vi "CRYGet BroadBand Curve.vi"(9 "Unit Info In":T5={"Y unit In"="dB", "dB ref In"=1.0, "Y unit Out"="dB", "dB ref Out"=1.0, "Y unit Curve"="dB", "dB ref Curve"=1.0, "Y data  Curve"=0, "Y data Time"=0}, 10 "Additive Info":T3, 11 "Impedance and Mic Current In":bool[](array[boolean])) -> (1 "Display Array":T4(array[cluster]), 2 "Unit Info Out":T2[](array[typedef]), 3 "Curve Info Array Out":T1)   [LabVIEW 2013]
uses:
  Typedef Control/CRYUnit Info Cluster.ctl
  Typedef Control/CRYUnit Info Out Cluster.ctl
  Typedef Control/CRYAnalysis CurveName Cluster.ctl
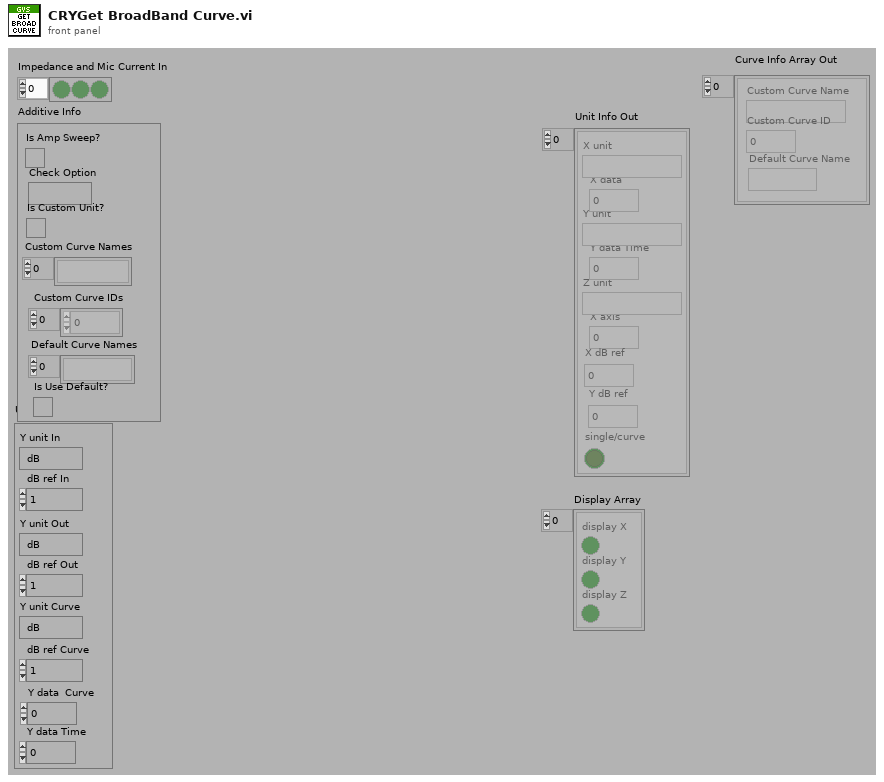
[diagram p1: front panel]
types:
  T1 = typedef "CRYAnalysis CurveName Cluster.ctl" = cluster{"Custom Curve Name":string, "Custom Curve ID":i32, "Default Curve Name":string}[]
  T2 = typedef "CRYUnit Info Out Cluster.ctl" = cluster{"X unit":string, "X data":u16, "Y unit":string, "Y data Time":u16, "Z unit":string, "X axis":u16, "X dB ref":dbl, "Y dB ref":dbl, "single/curve":bool}
  T3 = cluster{"Is Amp Sweep?":bool, "Check Option":string, "Is Custom Unit?":bool, "Custom Curve Names":string[], "Custom Curve IDs":i32[], "Default Curve Names":string[], "Is Use Default?":bool}
  T4 = cluster{"display X":bool, "display Y":bool, "display Z":bool}[]
  T5 = typedef "CRYUnit Info Cluster.ctl" = cluster{"Y unit In":string, "dB ref In":dbl, "Y unit Out":string, "dB ref Out":dbl, "Y unit Curve":string, "dB ref Curve":dbl, "Y data  Curve":u16, "Y data Time":u16}
  T6 = cluster{"display X":bool, "display Y":bool, "display Z":bool}
  T7 = enum32{"English", "Chinese", "Korean", "Japanese", "Russian", "Chinese traditional"}
  T8 = cluster{"Y unit Out":string, "dB":u16, "Y unit Curve":string, "Y data  Curve":u16, "Y unit Curve":string, "Lin":u16, "dB ref Out":dbl, "dB ref Curve":dbl, "display X":bool}
  T9 = cluster{"Y unit Out":string, "dB":u16, "Y unit Curve":string, "Y data  Curve":u16, "Y unit Curve":string, "Lin":u16, "dB ref Out":dbl, "dB ref Curve":dbl, "display X":bool}[]
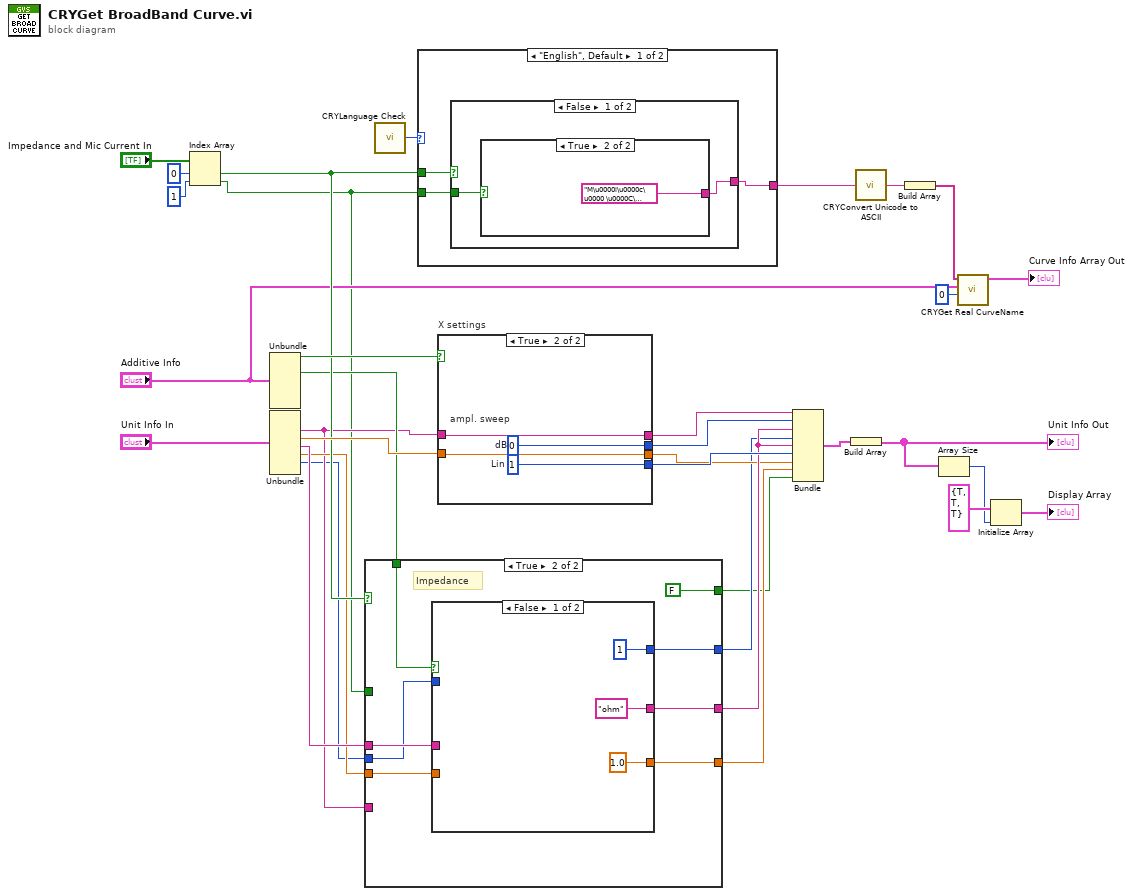
[diagram p0: block diagram]
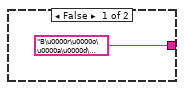
[diagram p2: hidden frame]
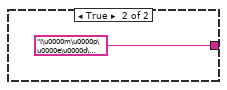
[diagram p3: hidden frame]
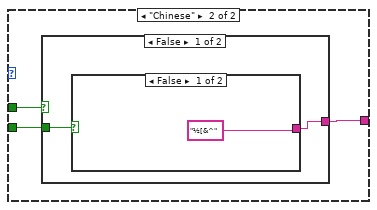
[diagram p4: hidden frame]
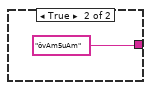
[diagram p5: hidden frame]
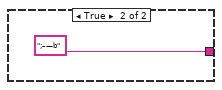
[diagram p6: hidden frame]
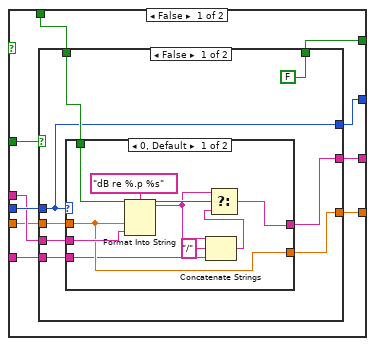
[diagram p7: hidden frame]
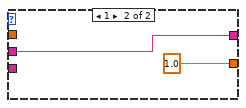
[diagram p8: hidden frame]
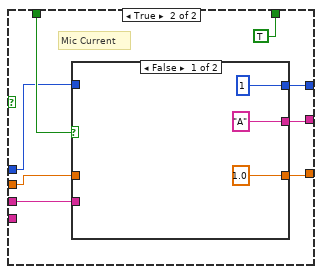
[diagram p9: hidden frame]
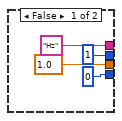
[diagram p12: hidden frame]
diagram:
  n1 = Index Array(array="Impedance and Mic Current In", index #1=0 ("index"), index #2=1 ("index")) -> (element #1=w27:bool, element #2=w4:bool)
  n2 = Unbundle("Additive Info") -> ("Is Amp Sweep?"=w30:bool, "Is Custom Unit?"=w13:bool)  [unwired: 5 out]
  n3 = Unbundle("Unit Info In") -> ("Y unit Out"=w12:string, "dB ref Out"=w29:dbl, "Y unit Curve"=w16:string, "dB ref Curve"=w15:dbl, "Y data  Curve"=w3:u16)  [unwired: 3 out]
  n4 = case shown="True" w27 {
    tunnel: w16 -> [w41 w81]
    tunnel: [w42 w84] -> w19
    tunnel: w3 -> [w43 w78]
    tunnel: w15 -> [w40 w80]
    tunnel: [w39 w83] -> w14
    tunnel: w13 -> [w38 w82]
    tunnel: w12 -> [w37 _]
    tunnel: w4 -> [w36 _]
    tunnel: [w35 w79] -> w2
    tunnel: [w34 FALSE ("display X")] -> w1
    frame False {
      n5 = case shown="False" w36 {
        tunnel: w43 -> [w45 w64]
        tunnel: [w51 w70] -> w42
        tunnel: w41 -> [w50 w66]
        tunnel: w40 -> [w49 w65]
        tunnel: [w48 w69] -> w39
        tunnel: w38 -> [w47 w68]
        tunnel: w37 -> [w46 _]
        tunnel: [w45 w67] -> w35
        tunnel: [FALSE ("display X") TRUE ("display X")] -> w34
        frame False {
          n6 = case shown="0, Default" w45 {
            tunnel: [w56 w61] -> w51
            tunnel: w49 -> [w59 _]
            tunnel: w50 -> [w60 w61]
            tunnel: [w59 1.0 ("dB ref Curve")] -> w48
            tunnel: w47 -> [w57 _]
            tunnel: w46 -> [w52 _]
            frame 0, Default {
              n7 = Format Into String(format string="dB re %.p %s", w59, w60) -> (resulting string=w54:string)  [unwired: 2 in, 1 out]
              n8 = Concatenate Strings(w54, "/" ("string"), w52) -> (w55:string)
              n9 = Select(t=w54, s=w57, f=w55) -> (s? t:f=w56:string)
            }
            frame 1 {
            }
          }
        }
        frame True {
          # "Mic Current"
          n10 = case shown="False" w68 {
            tunnel: ["A" ("unit") w75] -> w70
            tunnel: [1.0 ("dB ref Curve") w74] -> w69
            tunnel: [u16 1 ("Y data  Curve") w76] -> w67
            tunnel: w64 -> [_ w76]
            tunnel: w66 -> [_ w75]
            tunnel: w65 -> [_ w74]
            frame False {
            }
            frame True {
            }
          }
        }
      }
    }
    frame True {
      # "Impedance"
      n11 = case shown="False" w82 {
        tunnel: ["ohm" ("unit") w90] -> w84
        tunnel: [1.0 ("dB ref Curve") w89] -> w83
        tunnel: w81 -> [_ w90]
        tunnel: w80 -> [_ w89]
        tunnel: w78 -> [_ w88]
        tunnel: [u16 1 ("Y data  Curve") w88] -> w79
        frame False {
        }
        frame True {
        }
      }
    }
  }
  n12 = call "CRYLanguage Check.vi"() -> ("Language"=w5:T7)  [unwired: 10 in, 1 out]
  n13 = case shown="\"English\", Default" w5 {
    tunnel: w4 -> [w93 w101]
    tunnel: w27 -> [w92 w100]
    tunnel: [w91 w99] -> w6
    frame "English", Default {
      n14 = case shown="False" w92 {
        tunnel: w93 -> [w95 _]
        tunnel: [w94 "I\u0000m\u0000p\u0000e\u0000d\u0000a\u0000n\u0000c\u0000e\u0000" ("Unicode")] -> w91
        frame False {
          n15 = case shown="True" w95 {
            tunnel: ["B\u0000r\u0000o\u0000a\u0000d\u0000b\u0000a\u0000n\u0000d\u0000" ("message") "M\u0000i\u0000c\u0000 \u0000C\u0000u\u0000r\u0000r\u0000e\u0000n\u0000t\u0000" ("message")] -> w94
            frame False {
            }
            frame True {
            }
          }
        }
        frame True {
        }
      }
    }
    frame "Chinese" {
      n16 = case shown="False" w100 {
        tunnel: w101 -> [w103 _]
        tunnel: [w102 ";–—b" ("message")] -> w99
        frame False {
          n17 = case shown="False" w103 {
            tunnel: ["½[&^" ("message") "ôvAm5uAm" ("message")] -> w102
            frame False {
            }
            frame True {
            }
          }
        }
        frame True {
        }
      }
    }
  }
  n18 = case "X settings" shown="True" w30 {
    tunnel: ["Hz" ("X unit") w112] -> w22
    tunnel: [u16 1 ("Y data") w113] -> w21
    tunnel: [1.0 ("X dB ref") w111] -> w18
    tunnel: [u16 0 ("X axis") w114] -> w20
    tunnel: w12 -> [_ w112]
    tunnel: w29 -> [_ w111]
    frame False {
    }
    frame True {
      w113 = u16 0  # dB
      w114 = u16 1  # Lin
      # "ampl. sweep"
    }
  }
  n19 = Bundle("Y unit Out"=w22, "dB"=w21, "Y unit Curve"=w19, "Y data  Curve"=w2, "Y unit Curve"=w19, "Lin"=w20, "dB ref Out"=w18, "dB ref Curve"=w14, "display X"=w1) -> (w23:T8)  [unwired: 1 in]
  n20 = Build Array(w23) -> (w17:T9)
  "Unit Info Out" <- w17
  n21 = call "CRYConvert Unicode to ASCII.vi"("Unicode"=w6) -> ("ASCII"=w8:string)  [unwired: 4 in]
  n22 = Build Array(w8) -> (w7:string[])
  n23 = Array Size(array=w17) -> (size(s)=w25:i32)
  n24 = call "CRYGet Real CurveName.vi"("Key No"=0, "Additive Info"="Additive Info", "CurveArrayByType"=w7) -> ("Curve Info Array Out"=→"Curve Info Array Out":T1)  [unwired: 8 in]
  n25 = Initialize Array(T6 {"display X"=TRUE, "display Y"=TRUE, "display Z"=TRUE}, w25) -> (→"Display Array":T4)
